vi "Lab Panel V5.10.vi"() -> ()   [LabVIEW 2013] (continued)
                        n2910 = Build Path(base path=w5381, name or relative path="jigcycles.bin") -> (appended path=w5379:path)
                        n2911 = Create Folder(path (use dialog)=w5381) -> (error out=w5383:errorcluster)  [unwired: 2 in, 2 out]
                        n2912 = local read "JIG RELAY CYCLES"() -> (w5373:T8)
                        n2913 = call <vilib>:"Clear Errors.vi"("error in (no error)"=w5383) -> ()  [unwired: 6 in, 1 out]
                        n2914 = local write "Save JC"(FALSE) -> ()
                        n2915 = Open/Create/Replace File(file path (use dialog)=w5379, operation (0:open)=T21."replace or create") -> (refnum out=w5377:refnum<file>, error out=w5378:errorcluster)  [unwired: 4 in, 1 out]
                        n2916 = Write to Binary File(file (use dialog)=w5377, data=w5373, error in=w5378) -> (refnum out=w5376:refnum<file>, error out=w5375:errorcluster)  [unwired: 3 in, 1 out]
                        n2917 = Close File(refnum=w5376, error in=w5375) -> (error out=w5374:errorcluster)  [unwired: 1 out]
                        n2918 = local write "data file error"(w5374) -> ()
                      }
                      frame #1 {
                        n2919 = local read "JIG RELAY CYCLES"() -> (w5406:T8)
                        n2920 = Unbundle By Name(w5406) -> ("LAB01-1"=w5401:dbl, "LAB01-2"=w5400:dbl, "LAB02-1"=w5398:dbl, "LAB02-2"=w5397:dbl, "LAB03-1"=w5395:dbl, "LAB03-2"=w5392:dbl, "LAB04-1"=w5391:dbl, "LAB04-2"=w5389:dbl, "LAB05-1"=w5387:dbl, "LAB05-2"=w5385:dbl)
                        n2921 = stacked-sequence {
                          tunnel: w5401 -> [w5409 _ _ _ _ _ _ _ _ _]
                          tunnel: 1000000 -> [w5412 w5422 w5432 w5442 w5452 w5462 w5472 w5482 w5492 w5502]
                          tunnel: [w5410 _ _ _ _ _ _ _ _ _] -> w5404
                          tunnel: "TEST STATION HAS REACHED 1 MILLION CYCLES, REPLACE  CONTROL RELAYS" -> [w5408 w5420 w5430 w5440 w5450 w5460 w5470 w5480 w5490 w5500]
                          tunnel: [_ w5419 _ _ _ _ _ _ _ _] -> w5402
                          tunnel: w5400 -> [_ w5418 _ _ _ _ _ _ _ _]
                          tunnel: [_ _ w5429 _ _ _ _ _ _ _] -> w5399
                          tunnel: w5398 -> [_ _ w5428 _ _ _ _ _ _ _]
                          tunnel: w5397 -> [_ _ _ w5439 _ _ _ _ _ _]
                          tunnel: [_ _ _ w5438 _ _ _ _ _ _] -> w5396
                          tunnel: w5395 -> [_ _ _ _ w5449 _ _ _ _ _]
                          tunnel: [_ _ _ _ w5448 _ _ _ _ _] -> w5394
                          tunnel: [_ _ _ _ _ w5459 _ _ _ _] -> w5393
                          tunnel: w5392 -> [_ _ _ _ _ w5458 _ _ _ _]
                          tunnel: w5391 -> [_ _ _ _ _ _ w5469 _ _ _]
                          tunnel: [_ _ _ _ _ _ w5468 _ _ _] -> w5390
                          tunnel: w5389 -> [_ _ _ _ _ _ _ w5479 _ _]
                          tunnel: [_ _ _ _ _ _ _ w5478 _ _] -> w5388
                          tunnel: w5387 -> [_ _ _ _ _ _ _ _ w5489 _]
                          tunnel: [_ _ _ _ _ _ _ _ w5488 _] -> w5386
                          tunnel: w5385 -> [_ _ _ _ _ _ _ _ _ w5499]
                          tunnel: [_ _ _ _ _ _ _ _ _ w5498] -> w5384
                          frame #0 {
                            n2922 = Greater?(x=w5409, y=w5412) -> (0:w5411:bool)
                            n2923 = case shown="True" w5411 {
                              tunnel: [w5413 0] -> w5410
                              tunnel: w5409 -> [w5413 _]
                              tunnel: w5408 -> [_ w5414]
                              frame False {
                              }
                              frame True {
                                n2924 = Concatenate Strings("LA01-1 ", w5414) -> (w5417:string)
                                n2925 = One Button Dialog(message=w5417) -> ()  [unwired: 1 in, 1 out]
                              }
                            }
                          }
                          frame #1 {
                            n2926 = Greater?(x=w5418, y=w5422) -> (0:w5421:bool)
                            n2927 = case shown="True" w5421 {
                              tunnel: [w5423 0] -> w5419
                              tunnel: w5418 -> [w5423 _]
                              tunnel: w5420 -> [_ w5424]
                              frame False {
                              }
                              frame True {
                                n2928 = Concatenate Strings("LA01-2 ", w5424) -> (w5427:string)
                                n2929 = One Button Dialog(message=w5427) -> ()  [unwired: 1 in, 1 out]
                              }
                            }
                          }
                          frame #2 {
                            n2930 = Greater?(x=w5428, y=w5432) -> (0:w5431:bool)
                            n2931 = case shown="True" w5431 {
                              tunnel: [w5433 0] -> w5429
                              tunnel: w5428 -> [w5433 _]
                              tunnel: w5430 -> [_ w5434]
                              frame False {
                              }
                              frame True {
                                n2932 = Concatenate Strings("LA02-1 ", w5434) -> (w5437:string)
                                n2933 = One Button Dialog(message=w5437) -> ()  [unwired: 1 in, 1 out]
                              }
                            }
                          }
                          frame #3 {
                            n2934 = Greater?(x=w5439, y=w5442) -> (0:w5441:bool)
                            n2935 = case shown="True" w5441 {
                              tunnel: [w5443 0] -> w5438
                              tunnel: w5439 -> [w5443 _]
                              tunnel: w5440 -> [_ w5444]
                              frame False {
                              }
                              frame True {
                                n2936 = Concatenate Strings("LA02-2 ", w5444) -> (w5447:string)
                                n2937 = One Button Dialog(message=w5447) -> ()  [unwired: 1 in, 1 out]
                              }
                            }
                          }
                          frame #4 {
                            n2938 = Greater?(x=w5449, y=w5452) -> (0:w5451:bool)
                            n2939 = case shown="True" w5451 {
                              tunnel: [w5453 0] -> w5448
                              tunnel: w5449 -> [w5453 _]
                              tunnel: w5450 -> [_ w5454]
                              frame False {
                              }
                              frame True {
                                n2940 = Concatenate Strings("LA03-1 ", w5454) -> (w5457:string)
                                n2941 = One Button Dialog(message=w5457) -> ()  [unwired: 1 in, 1 out]
                              }
                            }
                          }
                          frame #5 {
                            n2942 = Greater?(x=w5458, y=w5462) -> (0:w5461:bool)
                            n2943 = case shown="True" w5461 {
                              tunnel: [w5463 0] -> w5459
                              tunnel: w5458 -> [w5463 _]
                              tunnel: w5460 -> [_ w5464]
                              frame False {
                              }
                              frame True {
                                n2944 = Concatenate Strings("LA03-2 ", w5464) -> (w5467:string)
                                n2945 = One Button Dialog(message=w5467) -> ()  [unwired: 1 in, 1 out]
                              }
                            }
                          }
                          frame #6 {
                            n2946 = Greater?(x=w5469, y=w5472) -> (0:w5471:bool)
                            n2947 = case shown="True" w5471 {
                              tunnel: [w5473 0] -> w5468
                              tunnel: w5469 -> [w5473 _]
                              tunnel: w5470 -> [_ w5474]
                              frame False {
                              }
                              frame True {
                                n2948 = Concatenate Strings("LA04-1 ", w5474) -> (w5477:string)
                                n2949 = One Button Dialog(message=w5477) -> ()  [unwired: 1 in, 1 out]
                              }
                            }
                          }
                          frame #7 {
                            n2950 = Greater?(x=w5479, y=w5482) -> (0:w5481:bool)
                            n2951 = case shown="True" w5481 {
                              tunnel: [w5483 0] -> w5478
                              tunnel: w5479 -> [w5483 _]
                              tunnel: w5480 -> [_ w5484]
                              frame False {
                              }
                              frame True {
                                n2952 = Concatenate Strings("LA04-2 ", w5484) -> (w5487:string)
                                n2953 = One Button Dialog(message=w5487) -> ()  [unwired: 1 in, 1 out]
                              }
                            }
                          }
                          frame #8 {
                            n2954 = Greater?(x=w5489, y=w5492) -> (0:w5491:bool)
                            n2955 = case shown="True" w5491 {
                              tunnel: [w5493 0] -> w5488
                              tunnel: w5489 -> [w5493 _]
                              tunnel: w5490 -> [_ w5494]
                              frame False {
                              }
                              frame True {
                                n2956 = Concatenate Strings("LA05-1 ", w5494) -> (w5497:string)
                                n2957 = One Button Dialog(message=w5497) -> ()  [unwired: 1 in, 1 out]
                              }
                            }
                          }
                          frame #9 {
                            n2958 = Greater?(x=w5499, y=w5502) -> (0:w5501:bool)
                            n2959 = case shown="True" w5501 {
                              tunnel: [w5503 0] -> w5498
                              tunnel: w5499 -> [w5503 _]
                              tunnel: w5500 -> [_ w5504]
                              frame False {
                              }
                              frame True {
                                n2960 = Concatenate Strings("LA05-2 ", w5504) -> (w5507:string)
                                n2961 = One Button Dialog(message=w5507) -> ()  [unwired: 1 in, 1 out]
                              }
                            }
                          }
                        }
                        n2962 = Bundle By Name(cluster=w5406, "LAB01-1"=w5404, "LAB01-2"=w5402, "LAB02-1"=w5399, "LAB02-2"=w5396, "LAB03-1"=w5394, "LAB03-2"=w5393, "LAB04-1"=w5390, "LAB04-2"=w5388, "LAB05-1"=w5386, "LAB05-2"=w5384) -> (w5405:T8)
                        n2963 = local write "JIG RELAY CYCLES"(w5405) -> ()
                      }
                    }
                  }
                }
              }
            }
          }
          frame #19 {
            # "get temperature values"
            n2964 = local read "Panel #"() -> (w5508:dbl)
            n2965 = local read "simulate"() -> (w5521:bool)
            n2966 = local read "Temp Test Cal"() -> (w5518:dbl)
            n2967 = stacked-sequence {
              seq-local: [w5524 _] -> [_ w5566]
              tunnel: w5521 -> [_ w5580]
              tunnel: T14 {"1  (A) cal"=1.0, "1 (V) cal"=1.0, "1 (PF) cal"=1.0, "1 (TL) cal"=1.0, "1 (TN) cal"=1.0, "2 (A) cal"=1.0, "2 (V) cal"=1.0, "2 (PF) cal"=1.0, "2 (TL) cal"=1.0, "2 (TN) cal"=1.0} ("CAL LAB01") -> [_ w5579]
              tunnel: w5519 -> [_ w5578]
              tunnel: w5518 -> [_ w5577]
              tunnel: w5517 -> [_ w5576]
              tunnel: w5516 -> [_ w5575]
              tunnel: w5515 -> [_ w5574]
              tunnel: w5514 -> [_ w5573]
              tunnel: w5513 -> [_ w5572]
              tunnel: w5512 -> [_ w5571]
              tunnel: w5511 -> [_ w5570]
              tunnel: w5510 -> [_ w5569]
              tunnel: w5509 -> [_ w5568]
              tunnel: w5508 -> [_ w5567]
              frame #0 {
                n2968 = local read "Select COM port"() -> (w5525:refnum<visa-resource-name>)
                "COM port" <- w5525
                n2969 = global write "Global 1.vi" "COM port"(w5525) -> ()
                n2970 = global write "Global 1.vi" "tmp dly lps"("Temp Delay Lps") -> ()
                n2971 = global write "Global 1.vi" "dly value"("Temp Value") -> ()
                n2972 = local read "jig cycle"() -> (w5527:dbl)
                n2973 = local read "on loops"() -> (w5529:dbl)
                n2974 = Add(x=w5529, y=3) -> (x+y=w5530:dbl)
                n2975 = local read "Panel #"() -> (w5526:dbl)
                n2976 = Equal?(x=w5527, y=w5530) -> (x = y?=w5524:bool)
                n2977 = case shown="True" w5524 {
                  tunnel: w5526 -> [_ w5534]
                  frame False {
                  }
                  frame True {
                    n2978 = local read "simulate"() -> (w5531:bool)
                    n2979 = case shown="1" w5534 {
                      tunnel: 1.0 -> [_ w5541 w5544 w5551 w5556 w5562]
                      tunnel: w5531 -> [_ w5537 w5543 w5549 w5557 w5561]
                      tunnel: [FALSE w5536 w5542 w5548 w5554 w5560] -> _
                      frame 0, Default {
                      }
                      frame 1 {
                        w5539 = FALSE
                        n2980 = call "sub vi - GET ALL TEMP v6.vi"("LA01-EN"=TRUE, "simulate"=w5537, "LA02-EN"=w5539, "LA03-EN"=w5539, "LA04-EN"=w5539, "LA05-EN"=w5539, "Gen Cal Value"=w5541) -> ("LA01 TEMP"=w5538:T24, "error"=w5536:bool)  [unwired: 3 in, 4 out]
                        n2981 = local write "LAB01 TEMP"(w5538) -> ()
                      }
                      frame 2 {
                        w5545 = FALSE
                        n2982 = call "sub vi - GET ALL TEMP v6.vi"("LA01-EN"=w5545, "simulate"=w5543, "LA02-EN"=TRUE, "LA03-EN"=w5545, "LA04-EN"=w5545, "LA05-EN"=w5545, "Gen Cal Value"=w5544) -> ("LA02 TEMP"=w5547:T24, "error"=w5542:bool)  [unwired: 3 in, 4 out]
                        n2983 = local write "LAB02 TEMP"(w5547) -> ()
                      }
                      frame 3 {
                        w5552 = FALSE
                        n2984 = call "sub vi - GET ALL TEMP v6.vi"("LA01-EN"=w5552, "simulate"=w5549, "LA02-EN"=w5552, "LA03-EN"=TRUE, "LA04-EN"=w5552, "LA05-EN"=w5552, "Gen Cal Value"=w5551) -> ("LA03 TEMP"=w5550:T24, "error"=w5548:bool)  [unwired: 3 in, 4 out]
                        n2985 = local write "LAB03 TEMP"(w5550) -> ()
                      }
                      frame 4 {
                        w5558 = FALSE
                        n2986 = call "sub vi - GET ALL TEMP v6.vi"("LA01-EN"=w5558, "simulate"=w5557, "LA02-EN"=w5558, "LA03-EN"=w5558, "LA04-EN"=TRUE, "LA05-EN"=w5558, "Gen Cal Value"=w5556) -> ("LA04 TEMP"=w5555:T24, "error"=w5554:bool)  [unwired: 3 in, 4 out]
                        n2987 = local write "LAB04 TEMP"(w5555) -> ()
                      }
                      frame 5 {
                        w5564 = FALSE
                        n2988 = call "sub vi - GET ALL TEMP v6.vi"("LA01-EN"=w5564, "simulate"=w5561, "LA02-EN"=w5564, "LA03-EN"=w5564, "LA04-EN"=w5564, "LA05-EN"=TRUE, "Gen Cal Value"=w5562) -> ("error"=w5560:bool, "LA05 TEMP"=w5563:T24)  [unwired: 3 in, 4 out]
                        n2989 = local write "LAB05 TEMP"(w5563) -> ()
                      }
                    }
                    n2990 = local write "TEMP"(TRUE) -> ()
                  }
                }
              }
              frame #1 {
                n2991 = case shown="True" w5566 {
                  tunnel: w5580 -> [_ w5594]
                  tunnel: w5579 -> [_ w5593]
                  tunnel: w5578 -> [_ w5592]
                  tunnel: w5577 -> [_ w5591]
                  tunnel: w5576 -> [_ w5590]
                  tunnel: w5575 -> [_ w5589]
                  tunnel: w5574 -> [_ w5588]
                  tunnel: w5573 -> [_ w5587]
                  tunnel: w5572 -> [_ w5586]
                  tunnel: w5571 -> [_ w5585]
                  tunnel: w5570 -> [_ w5584]
                  tunnel: w5569 -> [_ w5583]
                  tunnel: w5568 -> [_ w5582]
                  tunnel: w5567 -> [_ w5581]
                  frame False {
                  }
                  frame True {
                    n2992 = case shown="1" w5581 {
                      tunnel: w5594 -> [_ w5607 w5652 w5697 w5742 w5787]
                      tunnel: w5593 -> [_ w5606 w5651 w5696 w5741 w5786]
                      tunnel: w5592 -> [_ w5596 _ _ _ _]
                      tunnel: w5591 -> [_ w5601 w5650 w5695 w5740 w5785]
                      tunnel: w5590 -> [_ w5595 _ _ _ _]
                      tunnel: w5589 -> [_ _ w5641 _ _ _]
                      tunnel: w5588 -> [_ _ w5640 _ _ _]
                      tunnel: w5587 -> [_ _ _ w5686 _ _]
                      tunnel: w5586 -> [_ _ _ w5685 _ _]
                      tunnel: w5585 -> [_ _ _ _ w5731 _]
                      tunnel: w5584 -> [_ _ _ _ w5730 _]
                      tunnel: w5583 -> [_ _ _ _ _ w5776]
                      tunnel: w5582 -> [_ _ _ _ _ w5775]
                      frame ..0 {
                      }
                      frame 1 {
                        n2993 = case shown="False" w5607 {
                          tunnel: [w5638 w5639] -> w5623
                          tunnel: w5606 -> [_ w5639]
                          frame False {
                            n2994 = local read "CAL LAB01"() -> (w5638:T14)
                          }
                          frame True {
                          }
                        }
                        n2995 = local read "TEMP LA01"() -> (w5614:T9)
                        n2996 = local read "LAB01 TEMP"() -> (w5613:T12)
                        n2997 = call "sub vi - temperature delay v3.vi"("2-run"=w5595, "1-run"=w5596, "temp values IN"=w5614, "temp signals"=w5613) -> ("T2-N"=w5609:dbl, "T2-L"=w5610:dbl, "T1-N"=w5611:dbl, "T1-L"=w5612:dbl, "temp values OUT"=w5608:T43)  [unwired: 3 in]
                        n2998 = Unbundle By Name(w5623) -> ("1 (TL) cal"=w5618:dbl, "1 (TN) cal"=w5617:dbl, "2 (TL) cal"=w5616:dbl, "2 (TN) cal"=w5615:dbl)  [unwired: 6 out]
                        n2999 = local write "TEMP LA01"(w5608) -> ()
                        n3000 = Multiply(x=w5612, y=w5618) -> (x*y=w5605:dbl)
                        n3001 = Multiply(x=w5611, y=w5617) -> (x*y=w5603:dbl)
                        n3002 = Multiply(x=w5610, y=w5616) -> (x*y=w5600:dbl)
                        n3003 = Multiply(x=w5609, y=w5615) -> (x*y=w5599:dbl)
                        n3004 = case shown="True" w5596 {
                          tunnel: w5605 -> [w5632 w5637]
                          tunnel: w5601 -> [_ w5635]
                          tunnel: [w5632 w5636] -> w5604
                          tunnel: w5603 -> [w5631 w5634]
                          tunnel: [w5631 w5633] -> w5602
                          frame False {
                          }
                          frame True {
                            n3005 = Multiply(x=w5635, y=w5634) -> (x*y=w5633:dbl)
                            n3006 = Multiply(x=w5635, y=w5637) -> (x*y=w5636:dbl)
                          }
                        }
                        n3007 = case shown="True" w5595 {
                          tunnel: w5600 -> [w5625 w5630]
                          tunnel: w5601 -> [_ w5628]
                          tunnel: [w5625 w5629] -> w5598
                          tunnel: w5599 -> [w5624 w5627]
                          tunnel: [w5624 w5626] -> w5597
                          frame False {
                          }
                          frame True {
                            n3008 = Multiply(x=w5628, y=w5627) -> (x*y=w5626:dbl)
                            n3009 = Multiply(x=w5628, y=w5630) -> (x*y=w5629:dbl)
                          }
                        }
                        n3010 = local read "SIG LAB01-2"() -> (w5620:T2)
                        n3011 = local read "SIG LAB01-1"() -> (w5622:T2)
                        n3012 = Bundle By Name(cluster=w5622, "Tmp Live"=w5604, "Tmp Neut"=w5602) -> (w5621:T2)
                        n3013 = Bundle By Name(cluster=w5620, "Tmp Live"=w5598, "Tmp Neut"=w5597) -> (w5619:T2)
                        n3014 = local write "SIG LAB01-1"(w5621) -> ()
                        n3015 = local write "SIG LAB01-2"(w5619) -> ()
                      }
                      frame 2 {
                        n3016 = case shown="True" w5652 {
                          tunnel: [w5683 w5684] -> w5668
                          tunnel: w5651 -> [_ w5684]
                          frame False {
                            n3017 = local read "CAL LAB02"() -> (w5683:T15)
                          }
                          frame True {
                          }
                        }
                        n3018 = local read "LAB02 TEMP"() -> (w5659:T12)
                        n3019 = local read "TEMP LA02"() -> (w5658:T9)
                        n3020 = call "sub vi - temperature delay v3.vi"("2-run"=w5640, "1-run"=w5641, "temp values IN"=w5658, "temp signals"=w5659) -> ("T2-N"=w5653:dbl, "T2-L"=w5654:dbl, "T1-N"=w5655:dbl, "T1-L"=w5656:dbl, "temp values OUT"=w5657:T43)  [unwired: 3 in]
                        n3021 = Unbundle By Name(w5668) -> ("1 (TL) cal"=w5663:dbl, "1 (TN) cal"=w5662:dbl, "2 (TL) cal"=w5661:dbl, "2 (TN) cal"=w5660:dbl)  [unwired: 6 out]
                        n3022 = local write "TEMP LA02"(w5657) -> ()
                        n3023 = Multiply(x=w5656, y=w5663) -> (x*y=w5649:dbl)
                        n3024 = Multiply(x=w5655, y=w5662) -> (x*y=w5648:dbl)
                        n3025 = Multiply(x=w5654, y=w5661) -> (x*y=w5645:dbl)
                        n3026 = Multiply(x=w5653, y=w5660) -> (x*y=w5644:dbl)
                        n3027 = case shown="True" w5641 {
                          tunnel: w5649 -> [w5677 w5682]
                          tunnel: w5650 -> [_ w5680]
                          tunnel: [w5677 w5681] -> w5647
                          tunnel: w5648 -> [w5676 w5679]
                          tunnel: [w5676 w5678] -> w5646
                          frame False {
                          }
                          frame True {
                            n3028 = Multiply(x=w5680, y=w5679) -> (x*y=w5678:dbl)
                            n3029 = Multiply(x=w5680, y=w5682) -> (x*y=w5681:dbl)
                          }
                        }
                        n3030 = case shown="True" w5640 {
                          tunnel: w5645 -> [w5670 w5675]
                          tunnel: w5650 -> [_ w5673]
                          tunnel: [w5670 w5674] -> w5643
                          tunnel: w5644 -> [w5669 w5672]
                          tunnel: [w5669 w5671] -> w5642
                          frame False {
                          }
                          frame True {
                            n3031 = Multiply(x=w5673, y=w5672) -> (x*y=w5671:dbl)
                            n3032 = Multiply(x=w5673, y=w5675) -> (x*y=w5674:dbl)
                          }
                        }
                        n3033 = local read "SIG LAB02-2"() -> (w5665:T2)
                        n3034 = local read "SIG LAB02-1"() -> (w5667:T2)
                        n3035 = Bundle By Name(cluster=w5667, "Tmp Live"=w5647, "Tmp Neut"=w5646) -> (w5666:T2)
                        n3036 = Bundle By Name(cluster=w5665, "Tmp Live"=w5643, "Tmp Neut"=w5642) -> (w5664:T2)
                        n3037 = local write "SIG LAB02-1"(w5666) -> ()
                        n3038 = local write "SIG LAB02-2"(w5664) -> ()
                      }
                      frame 3 {
                        n3039 = case shown="False" w5697 {
                          tunnel: [w5728 w5729] -> w5713
                          tunnel: w5696 -> [_ w5729]
                          frame False {
                            n3040 = local read "CAL LAB03"() -> (w5728:T14)
                          }
                          frame True {
                          }
                        }
                        n3041 = local read "TEMP LA03"() -> (w5703:T9)
                        n3042 = local read "LAB03 TEMP"() -> (w5704:T12)
                        n3043 = call "sub vi - temperature delay v3.vi"("2-run"=w5685, "1-run"=w5686, "temp values IN"=w5703, "temp signals"=w5704) -> ("T2-N"=w5698:dbl, "T2-L"=w5699:dbl, "T1-N"=w5700:dbl, "T1-L"=w5701:dbl, "temp values OUT"=w5702:T43)  [unwired: 3 in]
                        n3044 = Unbundle By Name(w5713) -> ("1 (TL) cal"=w5708:dbl, "1 (TN) cal"=w5707:dbl, "2 (TL) cal"=w5706:dbl, "2 (TN) cal"=w5705:dbl)  [unwired: 6 out]
                        n3045 = local write "TEMP LA03"(w5702) -> ()
                        n3046 = Multiply(x=w5701, y=w5708) -> (x*y=w5694:dbl)
                        n3047 = Multiply(x=w5700, y=w5707) -> (x*y=w5693:dbl)
                        n3048 = Multiply(x=w5699, y=w5706) -> (x*y=w5690:dbl)
                        n3049 = Multiply(x=w5698, y=w5705) -> (x*y=w5689:dbl)
                        n3050 = case shown="True" w5685 {
                          tunnel: w5690 -> [w5715 w5720]
                          tunnel: w5695 -> [_ w5718]
                          tunnel: [w5715 w5719] -> w5688
                          tunnel: w5689 -> [w5714 w5717]
                          tunnel: [w5714 w5716] -> w5687
                          frame False {
                          }
                          frame True {
                            n3051 = Multiply(x=w5718, y=w5717) -> (x*y=w5716:dbl)
                            n3052 = Multiply(x=w5718, y=w5720) -> (x*y=w5719:dbl)
                          }
                        }
                        n3053 = case shown="True" w5686 {
                          tunnel: w5694 -> [w5722 w5727]
                          tunnel: w5695 -> [_ w5725]
                          tunnel: [w5722 w5726] -> w5692
                          tunnel: w5693 -> [w5721 w5724]
                          tunnel: [w5721 w5723] -> w5691
                          frame False {
                          }
                          frame True {
                            n3054 = Multiply(x=w5725, y=w5724) -> (x*y=w5723:dbl)
                            n3055 = Multiply(x=w5725, y=w5727) -> (x*y=w5726:dbl)
                          }
                        }
                        n3056 = local read "SIG LAB03-2"() -> (w5710:T2)
                        n3057 = local read "SIG LAB03-1"() -> (w5712:T2)
                        n3058 = Bundle By Name(cluster=w5712, "Tmp Live"=w5692, "Tmp Neut"=w5691) -> (w5711:T2)
                        n3059 = Bundle By Name(cluster=w5710, "Tmp Live"=w5688, "Tmp Neut"=w5687) -> (w5709:T2)
                        n3060 = local write "SIG LAB03-1"(w5711) -> ()
                        n3061 = local write "SIG LAB03-2"(w5709) -> ()
                      }
                      frame 4 {
                        n3062 = case shown="False" w5742 {
                          tunnel: [w5773 w5774] -> w5758
                          tunnel: w5741 -> [_ w5774]
                          frame False {
                            n3063 = local read "CAL LAB04"() -> (w5773:T14)
                          }
                          frame True {
                          }
                        }
                        n3064 = local read "LAB04 TEMP"() -> (w5748:T12)
                        n3065 = local read "TEMP LA04"() -> (w5749:T9)
                        n3066 = call "sub vi - temperature delay v3.vi"("2-run"=w5730, "1-run"=w5731, "temp values IN"=w5749, "temp signals"=w5748) -> ("T2-N"=w5743:dbl, "T2-L"=w5744:dbl, "T1-N"=w5745:dbl, "T1-L"=w5746:dbl, "temp values OUT"=w5747:T43)  [unwired: 3 in]
                        n3067 = Unbundle By Name(w5758) -> ("1 (TL) cal"=w5753:dbl, "1 (TN) cal"=w5752:dbl, "2 (TL) cal"=w5751:dbl, "2 (TN) cal"=w5750:dbl)  [unwired: 6 out]
                        n3068 = local write "TEMP LA04"(w5747) -> ()
                        n3069 = Multiply(x=w5746, y=w5753) -> (x*y=w5739:dbl)
                        n3070 = Multiply(x=w5745, y=w5752) -> (x*y=w5738:dbl)
                        n3071 = Multiply(x=w5744, y=w5751) -> (x*y=w5735:dbl)
                        n3072 = Multiply(x=w5743, y=w5750) -> (x*y=w5734:dbl)
                        n3073 = case shown="True" w5730 {
                          tunnel: w5735 -> [w5760 w5765]
                          tunnel: w5740 -> [_ w5763]
                          tunnel: [w5760 w5764] -> w5733
                          tunnel: w5734 -> [w5759 w5762]
                          tunnel: [w5759 w5761] -> w5732
                          frame False {
                          }
                          frame True {
                            n3074 = Multiply(x=w5763, y=w5762) -> (x*y=w5761:dbl)
                            n3075 = Multiply(x=w5763, y=w5765) -> (x*y=w5764:dbl)
                          }
                        }
                        n3076 = case shown="True" w5731 {
                          tunnel: w5739 -> [w5767 w5772]
                          tunnel: w5740 -> [_ w5770]
                          tunnel: [w5767 w5771] -> w5737
                          tunnel: w5738 -> [w5766 w5769]
                          tunnel: [w5766 w5768] -> w5736
                          frame False {
                          }
                          frame True {
                            n3077 = Multiply(x=w5770, y=w5769) -> (x*y=w5768:dbl)
                            n3078 = Multiply(x=w5770, y=w5772) -> (x*y=w5771:dbl)
                          }
                        }
                        n3079 = local read "SIG LAB04-2"() -> (w5755:T2)
                        n3080 = local read "SIG LAB04-1"() -> (w5757:T2)
                        n3081 = Bundle By Name(cluster=w5757, "Tmp Live"=w5737, "Tmp Neut"=w5736) -> (w5756:T2)
                        n3082 = Bundle By Name(cluster=w5755, "Tmp Live"=w5733, "Tmp Neut"=w5732) -> (w5754:T2)
                        n3083 = local write "SIG LAB04-1"(w5756) -> ()
                        n3084 = local write "SIG LAB04-2"(w5754) -> ()
                      }
                      frame 5.. {
                        n3085 = case shown="False" w5787 {
                          tunnel: [w5818 w5819] -> w5803
                          tunnel: w5786 -> [_ w5819]
                          frame False {
                            n3086 = local read "CAL LAB05"() -> (w5818:T14)
                          }
                          frame True {
                          }
                        }
                        n3087 = local read "LAB05 TEMP"() -> (w5793:T12)
                        n3088 = local read "TEMP LA05"() -> (w5794:T9)
                        n3089 = call "sub vi - temperature delay v3.vi"("2-run"=w5775, "1-run"=w5776, "temp values IN"=w5794, "temp signals"=w5793) -> ("T2-N"=w5789:dbl, "T2-L"=w5790:dbl, "T1-N"=w5791:dbl, "T1-L"=w5792:dbl, "temp values OUT"=w5788:T43)  [unwired: 3 in]
                        n3090 = local write "TEMP LA05"(w5788) -> ()
                        n3091 = Unbundle By Name(w5803) -> ("1 (TL) cal"=w5795:dbl, "1 (TN) cal"=w5798:dbl, "2 (TL) cal"=w5797:dbl, "2 (TN) cal"=w5796:dbl)  [unwired: 6 out]
                        n3092 = Multiply(x=w5792, y=w5795) -> (x*y=w5784:dbl)
                        n3093 = Multiply(x=w5791, y=w5798) -> (x*y=w5783:dbl)
                        n3094 = Multiply(x=w5790, y=w5797) -> (x*y=w5780:dbl)
                        n3095 = Multiply(x=w5789, y=w5796) -> (x*y=w5779:dbl)
                        n3096 = case shown="True" w5775 {
                          tunnel: w5780 -> [w5805 w5810]
                          tunnel: w5785 -> [_ w5808]
                          tunnel: [w5805 w5809] -> w5778
                          tunnel: w5779 -> [w5804 w5807]
                          tunnel: [w5804 w5806] -> w5777
                          frame False {
                          }
                          frame True {
                            n3097 = Multiply(x=w5808, y=w5807) -> (x*y=w5806:dbl)
                            n3098 = Multiply(x=w5808, y=w5810) -> (x*y=w5809:dbl)
                          }
                        }
                        n3099 = case shown="True" w5776 {
                          tunnel: w5784 -> [w5812 w5817]
                          tunnel: w5785 -> [_ w5815]
                          tunnel: [w5812 w5816] -> w5782
                          tunnel: w5783 -> [w5811 w5814]
                          tunnel: [w5811 w5813] -> w5781
                          frame False {
                          }
                          frame True {
                            n3100 = Multiply(x=w5815, y=w5814) -> (x*y=w5813:dbl)
                            n3101 = Multiply(x=w5815, y=w5817) -> (x*y=w5816:dbl)
                          }
                        }
                        n3102 = local read "SIG LAB05-1"() -> (w5802:T2)
                        n3103 = Bundle By Name(cluster=w5802, "Tmp Live"=w5782, "Tmp Neut"=w5781) -> (w5801:T2)
                        n3104 = local read "SIG LAB05-2"() -> (w5800:T2)
                        n3105 = Bundle By Name(cluster=w5800, "Tmp Live"=w5778, "Tmp Neut"=w5777) -> (w5799:T2)
                        n3106 = local write "SIG LAB05-1"(w5801) -> ()
                        n3107 = local write "SIG LAB05-2"(w5799) -> ()
                      }
                    }
                  }
                }
              }
            }
          }
          frame #20 {
            # "write data to display panel"
            n3108 = global write "Global display 1.vi" "TEST 5-2"(w5854) -> ()
            n3109 = global write "Global display 1.vi" "TEST 4-2"(w5856) -> ()
            n3110 = global write "Global display 1.vi" "TEST 1-2"(w5862) -> ()
            n3111 = global write "Global display 1.vi" "TEST 3-1"(w5859) -> ()
            n3112 = global write "Global display 1.vi" "TEST 5-1"(w5855) -> ()
            n3113 = global write "Global display 1.vi" "TEST 1-1"(w5863) -> ()
            n3114 = global write "Global display 1.vi" "TEST 3-2"(w5858) -> ()
            n3115 = global write "Global display 1.vi" "TEST 4-1"(w5857) -> ()
            n3116 = global write "Global display 1.vi" "TEST 2-2"(w5860) -> ()
            n3117 = global write "Global display 1.vi" "TEST 2-1"(w5861) -> ()
            n3118 = global read "Global display 3.vi" "log 1-1"() -> (→"LOG LAB01-1":string)
            n3119 = global read "Global display 3.vi" "log 3-1"() -> (→"LOG LAB03-1":string)
            n3120 = global read "Global display 3.vi" "log 1-2"() -> (→"LOG LAB01-2":string)
            n3121 = property on="Tab Control 2" class="TabCtl (strict)"() -> ("Pages"=w5853:refnum<vi>[])  [unwired: 2 in, 2 out]
            n3122 = global read "Global display 3.vi" "log 2-1"() -> (→"LOG LAB02-1":string)
            n3123 = global read "Global display 3.vi" "log 2-2"() -> (→"LOG LAB02-2":string)
            n3124 = global read "Global display 3.vi" "log 4-2"() -> (→"LOG LAB04-2":string)
            n3125 = global read "Global display 3.vi" "log 5-2"() -> (→"LOG LAB05-2":string)
            n3126 = global read "Global display 3.vi" "log 5-1"() -> (→"LOG LAB05-1":string)
            n3127 = global read "Global display 3.vi" "log 4-1"() -> (→"LOG LAB04-1":string)
            n3128 = global read "Global display 3.vi" "log 3-2"() -> (→"LOG LAB03-2":string)
            n3129 = Index Array(array=w5853, index=8) -> (element=w5851:refnum<vi>)
            n3130 = property class="Page"(reference=w5851) -> ("PageVis"=w5850:bool)  [unwired: 1 in, 2 out]
            n3131 = global write "Global display 3.vi" "admin"(w5850) -> ()
            n3132 = local read "O/I  LAB05-2"() -> (w5904:bool)
            n3133 = local read "O/I  LAB05-1"() -> (w5905:bool)
            n3134 = local read "O/I  LAB03-2"() -> (w5908:bool)
            n3135 = local read "O/I  LAB04-2"() -> (w5906:bool)
            n3136 = local read "O/I  LAB04-1"() -> (w5907:bool)
            n3137 = local read "O/I  LAB03-1"() -> (w5909:bool)
            n3138 = local read "O/I  LAB01-2"() -> (w5912:bool)
            n3139 = local read "O/I  LAB01-1"() -> (w5913:bool)
            n3140 = local read "O/I  LAB02-1"() -> (w5911:bool)
            n3141 = local read "O/I  LAB02-2"() -> (w5910:bool)
            n3142 = global write "Global display 1.vi" "5-2 O/F"(w5904) -> ()
            n3143 = global write "Global display 1.vi" "5-1 O/F"(w5905) -> ()
            n3144 = global write "Global display 1.vi" "4-1 O/F"(w5907) -> ()
            n3145 = global write "Global display 1.vi" "4-2 O/F"(w5906) -> ()
            n3146 = global write "Global display 1.vi" "3-2 O/F"(w5908) -> ()
            n3147 = global write "Global display 1.vi" "3-1 O/F"(w5909) -> ()
            n3148 = global write "Global display 1.vi" "2-2 O/F"(w5910) -> ()
            n3149 = global write "Global display 1.vi" "2-1 O/F"(w5911) -> ()
            n3150 = global write "Global display 1.vi" "1-2 O/F"(w5912) -> ()
            n3151 = global write "Global display 1.vi" "1-1 O/F"(w5913) -> ()
            n3152 = local read "TEMP START LAB02-2"() -> (w5836:cluster{"TL":dbl, "TN":dbl})
            n3153 = local read "run lab05-2"() -> (w5894:bool)
            n3154 = local read "TEMP START LAB01-2"() -> (w5838:cluster{"TL":dbl, "TN":dbl})
            n3155 = local read "TEMP START LAB02-1"() -> (w5837:cluster{"TL":dbl, "TN":dbl})
            n3156 = local read "TEMP START LAB04-1"() -> (w5833:cluster{"TL":dbl, "TN":dbl})
            n3157 = local read "TEMP START LAB04-2"() -> (w5832:cluster{"TL":dbl, "TN":dbl})
            n3158 = local read "run lab04-1"() -> (w5897:bool)
            n3159 = local read "run lab04-2"() -> (w5896:bool)
            n3160 = local read "run lab05-1"() -> (w5895:bool)
            n3161 = local read "TEMP START LAB01-1"() -> (w5839:cluster{"TL":dbl, "TN":dbl})
            n3162 = local read "TEMP START LAB05-2"() -> (w5830:cluster{"TL":dbl, "TN":dbl})
            n3163 = local read "TEMP START LAB05-1"() -> (w5831:cluster{"TL":dbl, "TN":dbl})
            n3164 = local read "run lab03-2"() -> (w5898:bool)
            n3165 = local read "TEMP START LAB03-2"() -> (w5834:cluster{"TL":dbl, "TN":dbl})
            n3166 = local read "TEMP START LAB03-1"() -> (w5835:cluster{"TL":dbl, "TN":dbl})
            n3167 = local read "run lab02-1"() -> (w5901:bool)
            n3168 = local read "run lab03-1"() -> (w5899:bool)
            n3169 = local read "run lab01-2"() -> (w5902:bool)
            n3170 = local read "run lab02-2"() -> (w5900:bool)
            n3171 = local read "run lab01-1"() -> (w5903:bool)
            n3172 = global write "Global display 1.vi" "5-2 R/S"(w5894) -> ()
            n3173 = global write "Global display 1.vi" "5-1 R/S"(w5895) -> ()
            n3174 = global write "Global display 1.vi" "4-2 R/S"(w5896) -> ()
            n3175 = global write "Global display 1.vi" "4-1 R/S"(w5897) -> ()
            n3176 = global write "Global display 1.vi" "3-2 R/S"(w5898) -> ()
            n3177 = global write "Global display 1.vi" "1-2 R/S"(w5902) -> ()
            n3178 = global write "Global display 1.vi" "2-1 R/S"(w5901) -> ()
            n3179 = global write "Global display 1.vi" "3-1 R/S"(w5899) -> ()
            n3180 = global write "Global display 1.vi" "2-2 R/S"(w5900) -> ()
            n3181 = global write "Global display 1.vi" "1-1 R/S"(w5903) -> ()
            n3182 = global write "Global display 3.vi" "TEMP ST 05-2"(w5830) -> ()
            n3183 = global write "Global display 3.vi" "TEMP ST 05-1"(w5831) -> ()
            n3184 = global write "Global display 3.vi" "TEMP ST 03-2"(w5834) -> ()
            n3185 = global write "Global display 3.vi" "TEMP ST 04-2"(w5832) -> ()
            n3186 = global write "Global display 3.vi" "TEMP ST 01-1"(w5839) -> ()
            n3187 = global write "Global display 3.vi" "TEMP ST 01-2"(w5838) -> ()
            n3188 = global write "Global display 3.vi" "TEMP ST 04-1"(w5833) -> ()
            n3189 = global write "Global display 3.vi" "TEMP ST 02-1"(w5837) -> ()
            n3190 = global write "Global display 3.vi" "TEMP ST 02-2"(w5836) -> ()
            n3191 = global write "Global display 3.vi" "TEMP ST 03-1"(w5835) -> ()
            n3192 = local read "DISP LAB04-2"() -> (w5886:T4)
            n3193 = local read "DISP LAB05-1"() -> (w5885:T4)
            n3194 = local read "DISP LAB04-1"() -> (w5887:T4)
            n3195 = local read "DISP LAB05-2"() -> (w5884:T4)
            n3196 = local read "DISP LAB03-1"() -> (w5889:T4)
            n3197 = local read "DISP LAB03-2"() -> (w5888:T4)
            n3198 = local read "DISP LAB01-2"() -> (w5892:T4)
            n3199 = local read "DISP LAB02-1"() -> (w5891:T4)
            n3200 = local read "DISP LAB02-2"() -> (w5890:T4)
            n3201 = local read "DISP LAB01-1"() -> (w5893:T4)
            n3202 = local read "TEMP RISE LAB05-1"() -> (w5821:cluster{"TL":dbl, "TN":dbl})
            n3203 = local read "TEMP RISE LAB05-2"() -> (w5820:cluster{"TL":dbl, "TN":dbl})
            n3204 = local read "TEMP RISE LAB04-2"() -> (w5822:cluster{"TL":dbl, "TN":dbl})
            n3205 = local read "TEMP RISE LAB04-1"() -> (w5823:cluster{"TL":dbl, "TN":dbl})
            n3206 = local read "TEMP RISE LAB03-2"() -> (w5824:cluster{"TL":dbl, "TN":dbl})
            n3207 = local read "TEMP RISE LAB03-1"() -> (w5825:cluster{"TL":dbl, "TN":dbl})
            n3208 = local read "TEMP RISE LAB01-2"() -> (w5828:cluster{"TL":dbl, "TN":dbl})
            n3209 = local read "TEMP RISE LAB02-2"() -> (w5826:cluster{"TL":dbl, "TN":dbl})
            n3210 = local read "TEMP RISE LAB01-1"() -> (w5829:cluster{"TL":dbl, "TN":dbl})
            n3211 = local read "TEMP RISE LAB02-1"() -> (w5827:cluster{"TL":dbl, "TN":dbl})
            n3212 = global write "Global display 2.vi" "DISP LAB05-1"(w5885) -> ()
            n3213 = global write "Global display 2.vi" "DISP LAB05-2"(w5884) -> ()
            n3214 = global write "Global display 2.vi" "DISP LAB04-2"(w5886) -> ()
            n3215 = global write "Global display 2.vi" "DISP LAB02-1"(w5891) -> ()
            n3216 = global write "Global display 2.vi" "DISP LAB02-2"(w5890) -> ()
            n3217 = global write "Global display 2.vi" "DISP LAB04-1"(w5887) -> ()
            n3218 = global write "Global display 2.vi" "DISP LAB01-2"(w5892) -> ()
            n3219 = global write "Global display 2.vi" "DISP LAB01-1"(w5893) -> ()
            n3220 = global write "Global display 2.vi" "DISP LAB03-1"(w5889) -> ()
            n3221 = global write "Global display 2.vi" "DISP LAB03-2"(w5888) -> ()
            n3222 = global write "Global display 3.vi" "TEMP RS 05-2"(w5820) -> ()
            n3223 = global write "Global display 3.vi" "TEMP RS 05-1"(w5821) -> ()
            n3224 = global write "Global display 3.vi" "TEMP RS 03-2"(w5824) -> ()
            n3225 = global write "Global display 3.vi" "TEMP RS 02-1"(w5827) -> ()
            n3226 = global write "Global display 3.vi" "TEMP RS 02-2"(w5826) -> ()
            n3227 = global write "Global display 3.vi" "TEMP RS 04-2"(w5822) -> ()
            n3228 = global write "Global display 3.vi" "TEMP RS 01-2"(w5828) -> ()
            n3229 = global write "Global display 3.vi" "TEMP RS 03-1"(w5825) -> ()
            n3230 = global write "Global display 3.vi" "TEMP RS 04-1"(w5823) -> ()
            n3231 = global write "Global display 3.vi" "TEMP RS 01-1"(w5829) -> ()
            n3232 = local read "SET LAB05-2"() -> (w5874:T5)
            n3233 = local read "SET LAB05-1"() -> (w5875:T5)
            n3234 = local read "SET LAB04-1"() -> (w5877:T5)
            n3235 = local read "SET LAB04-2"() -> (w5876:T5)
            n3236 = local read "SET LAB03-1"() -> (w5879:T5)
            n3237 = local read "SET LAB03-2"() -> (w5878:T5)
            n3238 = local read "SET LAB02-2"() -> (w5880:T5)
            n3239 = local read "SET LAB01-2"() -> (w5882:T5)
            n3240 = local read "SET LAB02-1"() -> (w5881:T5)
            n3241 = local read "SET LAB01-1"() -> (w5883:T5)
            n3242 = global write "Global display 2.vi" "SET LAB05-2"(w5874) -> ()
            n3243 = global write "Global display 2.vi" "SET LAB05-1"(w5875) -> ()
            n3244 = global write "Global display 2.vi" "SET LAB04-1"(w5877) -> ()
            n3245 = global write "Global display 2.vi" "SET LAB04-2"(w5876) -> ()
            n3246 = global write "Global display 2.vi" "SET LAB03-2"(w5878) -> ()
            n3247 = global write "Global display 2.vi" "SET LAB02-2"(w5880) -> ()
            n3248 = global write "Global display 2.vi" "SET LAB03-1"(w5879) -> ()
            n3249 = global write "Global display 2.vi" "SET LAB01-2"(w5882) -> ()
            n3250 = global write "Global display 2.vi" "SET LAB01-1"(w5883) -> ()
            n3251 = global write "Global display 2.vi" "SET LAB02-1"(w5881) -> ()
            n3252 = local read "RESULT LAB01-1"() -> (w5873:bool)
            n3253 = local read "RESULT LAB03-2"() -> (w5868:bool)
            n3254 = local read "RESULT LAB04-1"() -> (w5867:bool)
            n3255 = local read "RESULT LAB04-2"() -> (w5866:bool)
            n3256 = local read "RESULT LAB02-2"() -> (w5870:bool)
            n3257 = local read "RESULT LAB01-2"() -> (w5872:bool)
            n3258 = local read "RESULT LAB02-1"() -> (w5871:bool)
            n3259 = local read "RESULT LAB03-1"() -> (w5869:bool)
            n3260 = local read "RESULT LAB05-1"() -> (w5865:bool)
            n3261 = local read "RESULT LAB05-2"() -> (w5864:bool)
            n3262 = global write "Global display 2.vi" "RESULT LAB05-1"(w5865) -> ()
            n3263 = global write "Global display 2.vi" "RESULT LAB01-2"(w5872) -> ()
            n3264 = global write "Global display 2.vi" "RESULT LAB03-2"(w5868) -> ()
            n3265 = global write "Global display 2.vi" "RESULT LAB04-1"(w5867) -> ()
            n3266 = global write "Global display 2.vi" "RESULT LAB04-2"(w5866) -> ()
            n3267 = global write "Global display 2.vi" "RESULT LAB05-2"(w5864) -> ()
            n3268 = global write "Global display 2.vi" "RESULT LAB03-1"(w5869) -> ()
            n3269 = global write "Global display 2.vi" "RESULT LAB02-1"(w5871) -> ()
            n3270 = global write "Global display 2.vi" "RESULT LAB02-2"(w5870) -> ()
            n3271 = global write "Global display 2.vi" "RESULT LAB01-1"(w5873) -> ()
          }
          frame #21 {
            # "simulate values"
            n3272 = global write "Global display 4.vi" "LAB deg C"("LAB deg C") -> ()
          }
          frame #22 {
            # "end main and display program"
            n3273 = Quit LabVIEW(quit? (T)="stop all") -> ()
            n3274 = global write "Global display 1.vi" "stop disp"("stop all") -> ()
          }
        }
        n3275 = node-c288() -> ()  [unwired: 1 in, 1 out]
        "loops" <- w314
      }
      n3276 = node-c288(w291) -> ()  [unwired: 1 out]
    }
  }
